vi "FormatEvent.vi"(11 "EventData in":refnum<class "EventData.lvclass">) -> (3 "EventData out":refnum<class "EventData.lvclass">)   [LabVIEW 2016, in "Event Logging.lvlib" / "EventData.lvclass"]
uses:
  EventData.lvclass
  EventData.lvclass/EventData.ctl
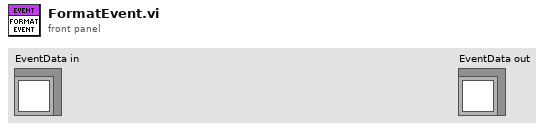
[diagram p1: front panel]
types:
  T1 = typedef "Event Logging.lvlib/EventData.lvclass/EventType.ctl" = enum16{"Event", "Warning", "Error"}
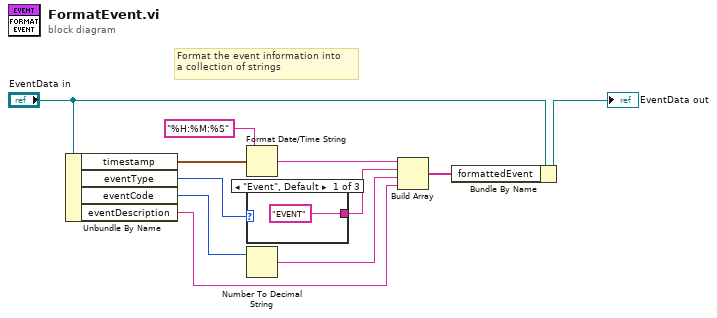
[diagram p0: block diagram]
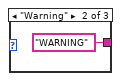
[diagram p2: hidden frame]
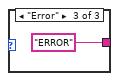
[diagram p3: hidden frame]
diagram:
  # "Format the event information into\na collection of strings"
  n1 = Unbundle By Name("EventData in") -> ("timestamp"=w11:timestamp, "eventType"=w9:T1, "eventCode"=w8:i32, "eventDescription"=w4:string)
  n2 = Format Date/Time String(time format string (%c)="%H:%M:%S", seconds (now)=w11) -> (date/time string=w7:string)  [unwired: 1 in]
  n3 = case shown="\"Event\", Default" w9 {
    tunnel: ["EVENT" "WARNING" "ERROR"] -> w6
    frame "Event", Default {
    }
    frame "Warning" {
    }
    frame "Error" {
    }
  }
  n4 = Number To Decimal String(number=w8) -> (decimal integer string=w5:string)  [unwired: 1 in]
  n5 = Build Array(w7, w6, w5, w4) -> (w3:string[])
  n6 = Bundle By Name(cluster="EventData in", "formattedEvent"=w3) -> (→"EventData out":refnum<class "EventData.lvclass">)
